vi "CheckPulses.vi"(7 "target pulses":i32, 9 "start index":i32, 10 "acquired pulses in":i32, 11 "DVR element in":T1) -> (1 "stop index (include)":i32, 2 "pulses met":bool, 4 "pulses":i32)   [LabVIEW 2017, in "DataAccumulator.lvlib"]
uses:
  <vilib>/addons/InsightCM/Devices/Shared/Common/DataAccumulator/DataAccumulator.lvlib
  <vilib>/addons/InsightCM/Devices/Shared/Common/DVRBuffer/controls/DVRElement.ctl
  <vilib>/addons/InsightCM/Devices/Shared/Common/DVRBuffer/DVRBuffer.lvlib
panel:
  # "if zero, use entire block"
  # "pulses contained in data from\nstart index to stop index.  if not\nenough pulses (stop index is 0),\nthis is the number of pulses in\ndata from start index through\nthe end of the block."
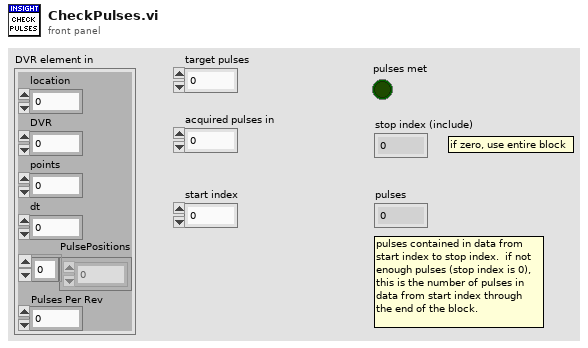
[diagram p1: front panel]
types:
  T1 = typedef "DVRBuffer.lvlib/DVRElement.ctl" = cluster{"location":u32, "DVR":u32, "points":i32, "dt":dbl, "PulsePositions":dbl[], "Pulses Per Rev":dbl}
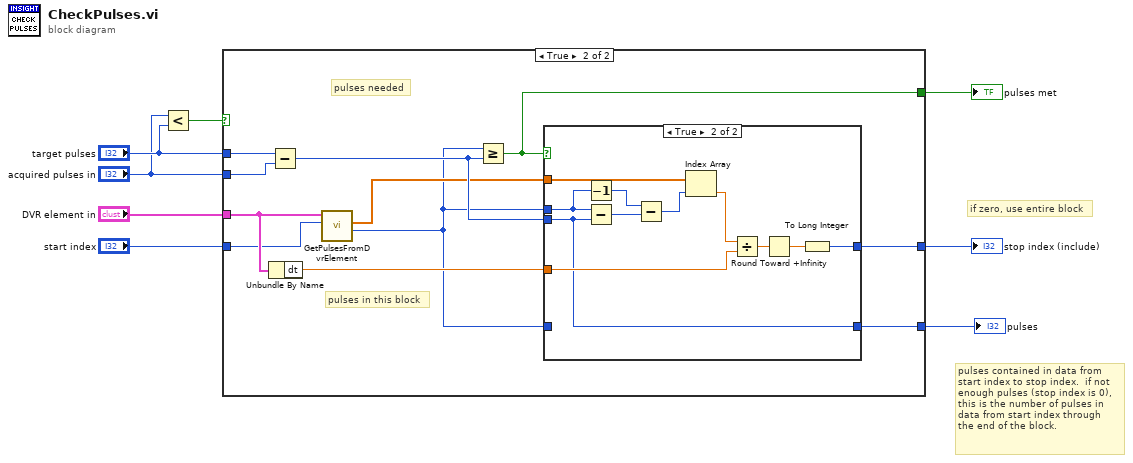
[diagram p0: block diagram]
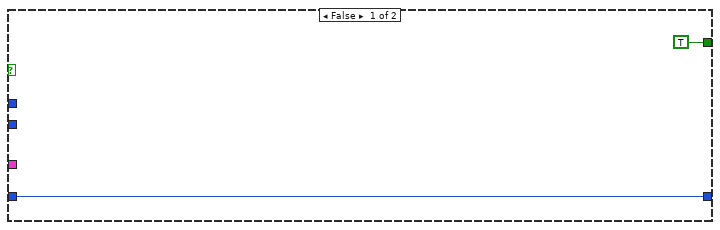
[diagram p2: hidden frame]
diagram:
  # "pulses contained in data from\nstart index to stop index.  if not\nenough pulses (stop index is 0),\nthis is the number of pulses in\ndata from start index through\nthe end of the block."
  # "if zero, use entire block"
  n1 = Less?(x="acquired pulses in", y="target pulses") -> (x < y?=w2:bool)
  n2 = case shown="True" w2 {
    tunnel: [TRUE w21] -> w8
    tunnel: "DVR element in" -> [_ w18]
    tunnel: "start index" -> [w9 w13]
    tunnel: [w9 w14] -> w5
    tunnel: "target pulses" -> [_ w16]
    tunnel: "acquired pulses in" -> [_ w15]
    tunnel: [_ w12] -> w1
    frame False {
    }
    frame True {
      # "pulses in this block"
      # "pulses needed"
      n3 = Unbundle By Name(w18) -> ("dt"=w19:dbl)
      n4 = Subtract(x=w16, y=w15) -> (x-y=w20:i32)
      n5 = call <vilib>:"GetPulsesFromDvrElement.vi"("index"=w13, "DVR element in"=w18) -> ("count"=w11:i32, "pulses"=w17:dbl[])  [unwired: 8 in]
      n6 = Greater Or Equal?(x=w11, y=w20) -> (x >= y?=w21:bool)
      n7 = case shown="True" w21 {
        tunnel: w11 -> [_ w30]
        tunnel: w19 -> [_ w31]
        tunnel: [_ w24] -> w14
        tunnel: w20 -> [_ w23]
        tunnel: w17 -> [_ w33]
        tunnel: [w22 w23] -> w12
        tunnel: w11 -> [w22 _]
        frame False {
          # "not enough pulses"
          # "Not enough points"
        }
        frame True {
          # "Too many points"
          n8 = Decrement(x=w30) -> (x-1=w29:i32)
          n9 = Subtract(x=w30, y=w23) -> (x-y=w28:i32)
          n10 = Subtract(x=w29, y=w28) -> (x-y=w27:i32)
          n11 = Index Array(array=w33, index=w27) -> (element=w32:dbl)
          n12 = Divide(x=w32, y=w31) -> (x/y=w26:dbl)
          n13 = Round Toward +Infinity(x=w26) -> (ceil(x): smallest int >= x=w25:dbl)
          n14 = To Long Integer(number=w25) -> (32bit integer=w24:i32)
        }
      }
    }
  }
  "pulses met" <- w8
  "stop index (include)" <- w5
  "pulses" <- w1
